vi "Main Analysis-Mechanical.vi"(0 "selected path":path, 5 "VI reference":refnum<vi>, 11 "Error In":errorcluster) -> (3 "error?":bool, 4 "Path out":path, 6 "PTP Array":dbl[](array[numeric]), 8 "SPL Array":dbl[](array[numeric]), 10 "SGP Array":dbl[](array[numeric]), 13 "F0 Array":dbl[](array[numeric]), 14 "Mean Flow (Overall)":dbl format="%0.3f", 15 "Error Out":errorcluster)   [LabVIEW 2020, in "MainVIs.lvlib"]
uses:
  MainVIs.lvlib
  AnalysisSupport.lvlib
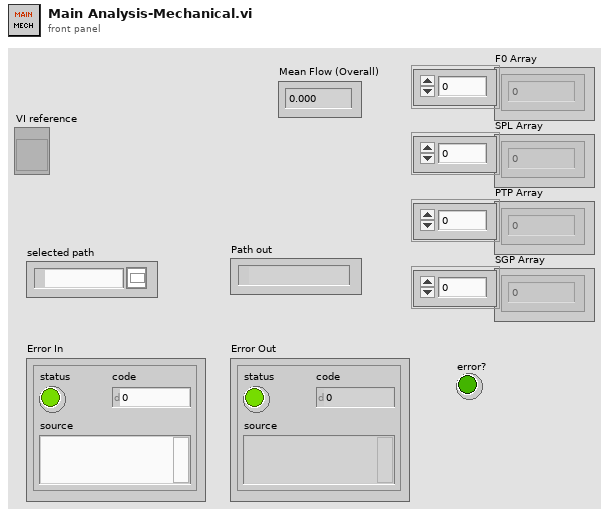
[diagram p1: front panel]
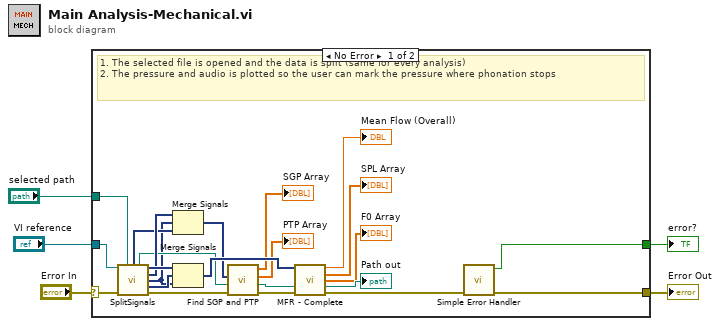
[diagram p0: block diagram]
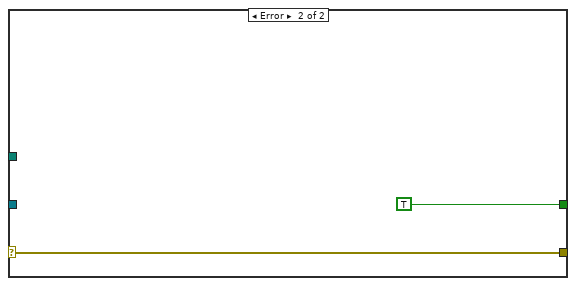
[diagram p2: hidden frame]
diagram:
  n1 = case shown="No Error" "Error In" {
    selector: "Error In" -> [w28 w29]
    tunnel: "selected path" -> [w27 _]
    tunnel: [w26 TRUE ("error?")] -> w3
    tunnel: [w25 w29] -> w2
    tunnel: "VI reference" -> [w20 _]
    frame No Error {
      # "1. The selected file is opened and the data is split (same for every analysis)\n2. The pressure and audio is plotted so the user can mark the pressure where phonation stops"
      n2 = call "SplitSignals.vi"("VI reference"=w20, "Filename"=w27, "Error In"=w28) -> ("EGG"=w15:dynamicdata, "Filename Out"=w13:path, "Flow"=w23:dynamicdata, "Pressure"=w16:dynamicdata, "Audio"=w7:dynamicdata, "SPL"=w22:dynamicdata, "Error Out"=w14:errorcluster)  [unwired: 5 in, 1 out]
      n3 = Merge Signals(w16, w7, w15) -> (w17:dynamicdata)
      n4 = Merge Signals(w23, w22, w7) -> (w21:dynamicdata)
      n5 = call "Find SGP and PTP.vi"("Error In"=w14, "File Path"=w13, "Pressure, Audio, EGG"=w17) -> ("Error Out"=w12:errorcluster, "File Path Indicator"=w9:path, "PTP Array"=→"PTP Array":dbl[], "SGP Array"=→"SGP Array":dbl[])  [unwired: 5 in]
      n6 = call "MFR - Complete.vi"("Flow, SPL & Audio"=w21, "File Name In"=w9, "Error In"=w12) -> ("Mean Flow (Overall)"=→"Mean Flow (Overall)":dbl, "SPL Array"=→"SPL Array":dbl[], "F0 Array"=→"F0 Array":dbl[], "File Name"=→"Path out":path, "Error Out"=w24:errorcluster)  [unwired: 8 in]
      n7 = call <vilib>:"Simple Error Handler.vi"("error in (no error)"=w24) -> ("error?"=w26:bool, "error out"=w25:errorcluster)  [unwired: 4 in, 3 out]
    }
    frame Error {
    }
  }
  "Error Out" <- w2
  "error?" <- w3
